vi "HFRR ADV v08.vi"() -> ()   [LabVIEW 2025] (continued)
                      frame #5 {
                        n2274 = local read "FILE"() -> (w3535:string)
                        n2275 = Concatenate Strings("File Name :" ("Content"), w3535) -> (w3536:string)
                        n2276 = local read "EVENT LOG"() -> (w3539:string)
                        n2277 = call "Event Log.vi"("Content"=w3536, "EVENT LOG"=w3539) -> ("EVENT LOG"=w3538:string)  [unwired: 8 in, 1 out]
                        n2278 = local write "EVENT LOG"(w3538) -> ()
                      }
                      frame #6 {
                        n2279 = Wait (ms)(milliseconds to wait=u32 50) -> ()  [unwired: 1 out]
                      }
                      frame #7 {
                        n2280 = local read "Batch Ref Num :"() -> (w3541:string)
                        n2281 = Concatenate Strings("Batch Ref No :" ("Content"), w3541) -> (w3542:string)
                        n2282 = local read "EVENT LOG"() -> (w3545:string)
                        n2283 = call "Event Log.vi"("Content"=w3542, "EVENT LOG"=w3545) -> ("EVENT LOG"=w3544:string)  [unwired: 8 in, 1 out]
                        n2284 = local write "EVENT LOG"(w3544) -> ()
                      }
                      frame #8 {
                        n2285 = Wait (ms)(milliseconds to wait=u32 50) -> ()  [unwired: 1 out]
                      }
                      frame #9 {
                        n2286 = local read "tested by"() -> (w3547:string)
                        n2287 = Concatenate Strings("Tested By :" ("Content"), w3547) -> (w3548:string)
                        n2288 = local read "EVENT LOG"() -> (w3551:string)
                        n2289 = call "Event Log.vi"("Content"=w3548, "EVENT LOG"=w3551) -> ("EVENT LOG"=w3550:string)  [unwired: 8 in, 1 out]
                        n2290 = local write "EVENT LOG"(w3550) -> ()
                      }
                      frame #10 {
                        n2291 = Wait (ms)(milliseconds to wait=u32 50) -> ()  [unwired: 1 out]
                      }
                      frame #11 {
                        n2292 = local read "TEST STANDARD"() -> (w3554:T4)
                        n2293 = case shown="\"ASTM D6079\", Default" w3554 {
                          tunnel: ["ASTM D6079" "ISO 12156" "CEC F-096-A-06" "Custom"] -> w3553
                          frame "ASTM D6079", Default {
                          }
                          frame "ISO 12156" {
                          }
                          frame "CEC F-096-A-06" {
                          }
                          frame "Custom" {
                          }
                        }
                        n2294 = Concatenate Strings("Test Standard :" ("Content"), w3553) -> (w3555:string)
                        n2295 = local read "EVENT LOG"() -> (w3558:string)
                        n2296 = call "Event Log.vi"("Content"=w3555, "EVENT LOG"=w3558) -> ("EVENT LOG"=w3557:string)  [unwired: 8 in, 1 out]
                        n2297 = local write "EVENT LOG"(w3557) -> ()
                      }
                      frame #12 {
                        n2298 = Wait (ms)(milliseconds to wait=u32 50) -> ()  [unwired: 1 out]
                      }
                      frame #13 {
                        n2299 = local read "Fuel Discription :"() -> (w3564:string)
                        n2300 = Concatenate Strings("Fuel Description :" ("Content"), w3564) -> (w3565:string)
                        n2301 = local read "EVENT LOG"() -> (w3568:string)
                        n2302 = call "Event Log.vi"("Content"=w3565, "EVENT LOG"=w3568) -> ("EVENT LOG"=w3567:string)  [unwired: 8 in, 1 out]
                        n2303 = local write "EVENT LOG"(w3567) -> ()
                      }
                      frame #14 {
                        n2304 = Wait (ms)(milliseconds to wait=u32 50) -> ()  [unwired: 1 out]
                      }
                      frame #15 {
                        n2305 = local read "Remarks :"() -> (w3570:string)
                        n2306 = Concatenate Strings("Remarks :" ("Content"), w3570) -> (w3571:string)
                        n2307 = local read "EVENT LOG"() -> (w3574:string)
                        n2308 = call "Event Log.vi"("Content"=w3571, "EVENT LOG"=w3574) -> ("EVENT LOG"=w3573:string)  [unwired: 8 in, 1 out]
                        n2309 = local write "EVENT LOG"(w3573) -> ()
                      }
                      frame #16 {
                        n2310 = Wait (ms)(milliseconds to wait=u32 50) -> ()  [unwired: 1 out]
                      }
                      frame #17 {
                        n2311 = local read "Operator ID"() -> (w3576:string)
                        n2312 = Concatenate Strings("Operator ID :" ("Content"), w3576) -> (w3578:string)
                        n2313 = local read "EVENT LOG"() -> (w3580:string)
                        n2314 = call "Event Log.vi"("Content"=w3578, "EVENT LOG"=w3580) -> ("EVENT LOG"=w3579:string)  [unwired: 8 in, 1 out]
                        n2315 = local write "EVENT LOG"(w3579) -> ()
                      }
                      frame #18 {
                        n2316 = Wait (ms)(milliseconds to wait=u32 50) -> ()  [unwired: 1 out]
                      }
                      frame #19 {
                        n2317 = disable-structure shown="Disabled" {
                          frame Disabled {
                            n2318 = local read "EVENT LOG"() -> (w3584:string)
                            n2319 = call "Event Log.vi"("Content"="Test Parameter", "EVENT LOG"=w3584) -> ("EVENT LOG"=w3583:string)  [unwired: 8 in, 1 out]
                            n2320 = local write "EVENT LOG"(w3583) -> ()
                          }
                          frame Enabled {
                          }
                        }
                      }
                      frame #20 {
                        n2321 = Wait (ms)(milliseconds to wait=u32 50) -> ()  [unwired: 1 out]
                      }
                      frame #21 {
                        n2322 = local read "Set Hz"() -> (w3588:dbl)
                        n2323 = Number To Fractional String(number=w3588, precision (6)=i16 2) -> (F-format string=w3587:string)  [unwired: 2 in]
                        n2324 = Concatenate Strings("Set Frequency [Hz] :" ("Content"), w3587) -> (w3590:string)
                        n2325 = local read "EVENT LOG"() -> (w3592:string)
                        n2326 = call "Event Log.vi"("Content"=w3590, "EVENT LOG"=w3592) -> ("EVENT LOG"=w3591:string)  [unwired: 8 in, 1 out]
                        n2327 = local write "EVENT LOG"(w3591) -> ()
                      }
                      frame #22 {
                        n2328 = Wait (ms)(milliseconds to wait=u32 50) -> ()  [unwired: 1 out]
                      }
                      frame #23 {
                        n2329 = local read "NORMAL LOAD"() -> (w3595:dbl)
                        n2330 = Number To Fractional String(number=w3595, precision (6)=i16 2) -> (F-format string=w3596:string)  [unwired: 2 in]
                        n2331 = Concatenate Strings("Applied Load [N] :" ("Content"), w3596) -> (w3598:string)
                        n2332 = local read "EVENT LOG"() -> (w3600:string)
                        n2333 = call "Event Log.vi"("Content"=w3598, "EVENT LOG"=w3600) -> ("EVENT LOG"=w3599:string)  [unwired: 8 in, 1 out]
                        n2334 = local write "EVENT LOG"(w3599) -> ()
                      }
                      frame #24 {
                        n2335 = Wait (ms)(milliseconds to wait=u32 50) -> ()  [unwired: 1 out]
                      }
                      frame #25 {
                        n2336 = local read "Set Strk"() -> (w3603:dbl)
                        n2337 = Number To Fractional String(number=w3603, precision (6)=i16 2) -> (F-format string=w3604:string)  [unwired: 2 in]
                        n2338 = Concatenate Strings("Set Stroke [mm] :" ("Content"), w3604) -> (w3606:string)
                        n2339 = local read "EVENT LOG"() -> (w3608:string)
                        n2340 = call "Event Log.vi"("Content"=w3606, "EVENT LOG"=w3608) -> ("EVENT LOG"=w3607:string)  [unwired: 8 in, 1 out]
                        n2341 = local write "EVENT LOG"(w3607) -> ()
                      }
                      frame #26 {
                        n2342 = Wait (ms)(milliseconds to wait=u32 50) -> ()  [unwired: 1 out]
                      }
                      frame #27 {
                        n2343 = local read "Set Temp"() -> (w3611:dbl)
                        n2344 = Number To Fractional String(number=w3611, precision (6)=i16 2) -> (F-format string=w3612:string)  [unwired: 2 in]
                        n2345 = Concatenate Strings("Set Temperature [deg C] :" ("Content"), w3612) -> (w3614:string)
                        n2346 = local read "EVENT LOG"() -> (w3616:string)
                        n2347 = call "Event Log.vi"("Content"=w3614, "EVENT LOG"=w3616) -> ("EVENT LOG"=w3615:string)  [unwired: 8 in, 1 out]
                        n2348 = local write "EVENT LOG"(w3615) -> ()
                      }
                      frame #28 {
                        n2349 = Wait (ms)(milliseconds to wait=u32 50) -> ()  [unwired: 1 out]
                      }
                      frame #29 {
                        n2350 = local read "Set Rh"() -> (w3619:dbl)
                        n2351 = Number To Fractional String(number=w3619, precision (6)=i16 2) -> (F-format string=w3620:string)  [unwired: 2 in]
                        n2352 = Concatenate Strings("Set Humidity [%RH] :" ("Content"), w3620) -> (w3622:string)
                        n2353 = local read "EVENT LOG"() -> (w3624:string)
                        n2354 = call "Event Log.vi"("Content"=w3622, "EVENT LOG"=w3624) -> ("EVENT LOG"=w3623:string)  [unwired: 8 in, 1 out]
                        n2355 = local write "EVENT LOG"(w3623) -> ()
                      }
                      frame #30 {
                        n2356 = Wait (ms)(milliseconds to wait=u32 50) -> ()  [unwired: 1 out]
                      }
                      frame #31 {
                        n2357 = local read "test time"() -> (w3627:dbl)
                        n2358 = Number To Fractional String(number=w3627, precision (6)=i16 1) -> (F-format string=w3628:string)  [unwired: 2 in]
                        n2359 = Concatenate Strings("Test Duration [mins] :" ("Content"), w3628) -> (w3630:string)
                        n2360 = local read "EVENT LOG"() -> (w3632:string)
                        n2361 = call "Event Log.vi"("Content"=w3630, "EVENT LOG"=w3632) -> ("EVENT LOG"=w3631:string)  [unwired: 8 in, 1 out]
                        n2362 = local write "EVENT LOG"(w3631) -> ()
                      }
                    }
                  }
                }
              }
            }
          }
        }
        n2363 = case shown="True" w2930 {
          frame False {
            n2364 = local write "tfalg"(0.0 ("tfalg")) -> ()
          }
          frame True {
            n2365 = local read "tfalg"() -> (w3075:dbl)
            n2366 = Equal?(x=w3075, y=0.0) -> (x = y?=w3076:bool)
            n2367 = case shown="True" w3076 {
              frame False {
              }
              frame True {
                n2368 = local read "Total No. of Tests"() -> (w3079:dbl)
                n2369 = local write "tfalg"(1.0 ("tfalg")) -> ()
                n2370 = local write "acq 2"(FALSE ("acq 2")) -> ()
                n2371 = Wait (ms)(milliseconds to wait=u32 200) -> ()  [unwired: 1 out]
                n2372 = Increment(x=w3079) -> (x+1=w3078:dbl)
                n2373 = local write "Total No. of Tests"(w3078) -> ()
              }
            }
          }
        }
        n2374 = local write "Test \nStatus"(w2936) -> ()
        n2375 = local write "st enable"(w2936) -> ()
        n2376 = local write "PWR"(w2936) -> ()
        n2377 = local write "Save"(w2936) -> ()
        n2378 = local read "Main Tab"() -> (w2893:T3)
        n2379 = case shown="True" w2917 {
          tunnel: [FALSE ("RUN") TRUE ("RUN")] -> w2916
          tunnel: [_ 1] -> w2909
          frame False {
          }
          frame True {
          }
        }
        n2380 = In Range and Coerce(upper limit=w2924, x=w2897, lower limit=w2923) -> (In Range?=w2915:bool)  [unwired: 1 out]
        n2381 = In Range and Coerce(upper limit=w2921, x=w2896, lower limit=w2922) -> (In Range?=w2913:bool)  [unwired: 1 out]
        n2382 = case shown="True" w2929 {
          frame False {
            n2383 = local read "Rt 3"() -> (w3057:bool)
            n2384 = case shown="True" w3057 {
              frame False {
              }
              frame True {
                n2385 = local write "Rt 3"(FALSE ("Rt 3")) -> ()
                n2386 = local write "Json End Flg"(TRUE ("Upld AR 2")) -> ()
              }
            }
            "Rt" <- TRUE ("Rt")
            "Rt 2" <- FALSE ("Rt")
          }
          frame True {
            n2387 = local read "Rt"() -> (w3064:bool)
            n2388 = local write "Rt 2"(TRUE ("Rt 2")) -> ()
            n2389 = case shown="True" w3064 {
              frame False {
              }
              frame True {
                w3065 = TRUE ("Upld AR 2")
                n2390 = local write "Rt"(FALSE ("Rt")) -> ()
                n2391 = local write "Upld AR"(w3065) -> ()
                n2392 = local write "Json St Flg"(w3065) -> ()
              }
            }
            "Rt 3" <- TRUE ("Rt 3")
          }
        }
        n2393 = case shown="True" w2915 {
          tunnel: [FALSE ("RUN") TRUE ("RUN")] -> w2914
          tunnel: [_ 2] -> w2908
          frame False {
          }
          frame True {
          }
        }
        n2394 = case shown="True" w2913 {
          tunnel: [FALSE ("RUN") TRUE ("RUN")] -> w2912
          tunnel: [_ 3] -> w2907
          frame False {
          }
          frame True {
          }
        }
        n2395 = case shown="\"Acquire\"" w2893 {
          tunnel: w2895 -> [_ w3126]
          frame Default {
            w3125 = 0.0 ("output")
            n2396 = local write "PID-out"(w3125) -> ()
            n2397 = local write "Frequency ( Hz )"(w3125) -> ()
          }
          frame "Acquire" {
            n2398 = stacked-sequence {
              frame #0 {
                n2399 = local read "Auto Start Test"() -> (w3128:bool)
                n2400 = case shown="False" w3128 {
                  tunnel: "RUN" -> [w3149 w3152]
                  tunnel: [w3149 w3151] -> w3129
                  frame False {
                  }
                  frame True {
                    n2401 = local read "Auto Start Temp"() -> (w3150:bool)
                    n2402 = Or(x=w3152, y=w3150) -> (x .or. y?=w3151:bool)
                  }
                }
                n2403 = local read "clk"() -> (w3148:dbl)
                n2404 = local read "Save"() -> (w3144:bool)
                n2405 = Equal?(x=w3148, y=0.0) -> (x = y?=w3145:bool)
                n2406 = And(x=w3145, y=w3144) -> (x .and. y?=w3146:bool)
                n2407 = Not(x="Engage") -> (.not. x?=w3135:bool)
                n2408 = case shown="True" w3129 {
                  tunnel: [w3160 w3178] -> w3131
                  frame False {
                    w3160 = 0.0
                    n2409 = local read "Auto Start Test"() -> (w3156:bool)
                    n2410 = local write "Reinit PID"(TRUE) -> ()
                    n2411 = local write "Start Time"(TRUE ("Start Time")) -> ()
                    n2412 = property on="Stroke" class="DigNum (strict)"("Visible"=TRUE) -> ()  [unwired: 2 in, 2 out]
                    n2413 = property on="Stroke 2" class="DigNum (strict)"("Visible"=FALSE) -> ()  [unwired: 2 in, 2 out]
                    n2414 = case shown="False" w3156 {
                      frame False {
                        n2415 = property on="Heater Button" class="Bool (strict)"("DisabledEnum"=T15."Enabled" ("Disabled")) -> ()  [unwired: 2 in, 2 out]
                        n2416 = property on="Humidity" class="Bool (strict)"("DisabledEnum"=T15."Enabled" ("Disabled")) -> ()  [unwired: 2 in, 2 out]
                      }
                      frame True {
                      }
                    }
                    n2417 = case shown="False" "TestCompFlg" {
                      frame False {
                        n2418 = local read "StartFlg"() -> (w3166:bool)
                        n2419 = case shown="True" w3166 {
                          frame False {
                          }
                          frame True {
                            n2420 = flat-sequence {
                              frame #0 {
                                n2421 = local read "EVENT LOG"() -> (w3168:string)
                                n2422 = call "Event Log.vi"("Content"="Test was interrupted", "EVENT LOG"=w3168) -> ("EVENT LOG"=w3169:string)  [unwired: 8 in, 1 out]
                                n2423 = local write "EVENT LOG"(w3169) -> ()
                              }
                              frame #1 {
                                w3170 = FALSE ("StartFlg")
                                n2424 = local write "Heater Button"(w3170) -> ()
                                n2425 = local write "StartFlg"(w3170) -> ()
                                n2426 = local write "Humidity"(w3170) -> ()
                              }
                            }
                          }
                        }
                      }
                      frame True {
                      }
                    }
                    n2427 = local write "String 14"("Test will autostart once parameters reach the set value." ("String 14")) -> ()
                    n2428 = local write "Old Pid Val"(w3160) -> ()
                  }
                  frame True {
                    n2429 = property on="Stroke 2" class="DigNum (strict)"("Visible"=TRUE) -> ()  [unwired: 2 in, 2 out]
                    n2430 = property on="Stroke" class="DigNum (strict)"("Visible"=FALSE) -> ()  [unwired: 2 in, 2 out]
                    n2431 = property on="STOP 2" class="Bool (strict)"("Disabled"=u8 2) -> ()  [unwired: 2 in, 2 out]
                    n2432 = local write "String 14"(" Running....." ("String 14")) -> ()
                    n2433 = property on="Heater Button" class="Bool (strict)"("DisabledEnum"=T15."Disabled and Grayed Out" ("Disabled")) -> ()  [unwired: 2 in, 2 out]
                    n2434 = property on="Humidity" class="Bool (strict)"("DisabledEnum"=T15."Disabled and Grayed Out" ("Disabled")) -> ()  [unwired: 2 in, 2 out]
                    n2435 = local read "PID Ref"() -> (w3189:bool)
                    n2436 = case shown="True" w3189 {
                      tunnel: [w3195 w3211] -> w3188
                      frame False {
                        n2437 = local read "Old Pid Val"() -> (w3195:dbl)
                      }
                      frame True {
                        n2438 = local read "Set Hz"() -> (w3204:dbl)
                        n2439 = local read "Frequency"() -> (w3215:dbl)
                        n2440 = Add(x=w3204, y=10.0) -> (x+y=w3213:dbl)
                        n2441 = Add(x=w3204, y=-10.0 ("Offset")) -> (x+y=w3222:dbl)
                        n2442 = Add(x=w3204, y=-10.0) -> (x+y=w3214:dbl)
                        n2443 = In Range and Coerce(upper limit=w3213, x=w3215, lower limit=w3214) -> (coerced(x)=w3203:dbl)  [unwired: 1 out]
                        n2444 = Or(x="Reinit PID", y="Reinit PID") -> (x .or. y?=w3212:bool)
                        n2445 = Multiply(x=w3222, y=0.1 ("Gain")) -> (x*y=w3201:dbl)
                        n2446 = local read "Elapsed time"() -> (w3208:dbl)
                        n2447 = local read "SPEED OUT:"() -> (w3223:dbl)
                        n2448 = Add(x=w3201, y=1.5) -> (x+y=w3199:dbl)
                        n2449 = call-poly <vilib>:"PID.vi"("reinitialize? (F)"=w3212, "output range"=cluster{"output high":dbl, "output low":dbl} {"output high"=1.0, "output low"=-1.0}, "PID gains"=T11 {"proportional gain (Kc)"=0.0005, "integral time (Ti, min)"=0.001, "derivative time (Td, min)"=0.0} ("Motor PID"), "process variable"=w3203, "setpoint"=w3204) -> ("output"=w3202:dbl)  [unwired: 5 in, 1 out]
                        n2450 = Multiply(x=w3199, y=w3223) -> (x*y=w3198:dbl)
                        n2451 = Greater?(x=w3208, y=0.05) -> (0:w3207:bool)
                        n2452 = case shown="True" w3207 {
                          tunnel: w3202 -> [_ w3225]
                          tunnel: [0.0 ("output") w3225] -> w3205
                          frame False {
                          }
                          frame True {
                            n2453 = local write "Reinit PID"(FALSE ("Reinit PID")) -> ()
                          }
                        }
                        n2454 = Multiply(x=w3198, y=0.8) -> (x*y=w3197:dbl)
                        n2455 = Add(x=w3197, y=w3205) -> (x+y=w3210:dbl)
                        n2456 = flat-sequence {
                          tunnel: [w3228] -> w3211
                          tunnel: w3210 -> [w3228]
                          frame #0 {
                            n2457 = local write "PID Ref"(FALSE ("PID Ref")) -> ()
                          }
                        }
                      }
                    }
                    "Old Pid Val" <- w3188
                    n2458 = case shown="False" "Start Time" {
                      selector: "Start Time" -> [_ w3191]
                      frame False {
                      }
                      frame True {
                        n2459 = Not(x=w3191) -> (.not. x?=w3190:bool)
                        n2460 = local write "Start Time"(w3190) -> ()
                        n2461 = local read "EVENT LOG"() -> (w3192:string)
                        n2462 = call "Event Log.vi"("Content"="Test in progress", "EVENT LOG"=w3192) -> ("EVENT LOG"=w3194:string)  [unwired: 8 in, 1 out]
                        n2463 = local write "EVENT LOG"(w3194) -> ()
                      }
                    }
                    n2464 = local read "Set Hz"() -> (w3185:dbl)
                    n2465 = call <vilib>:"Uniform White Noise Waveform.vi"() -> ("signal out"=w3184:waveform(dbl))  [unwired: 10 in, 1 out]
                    n2466 = local read "Freq"() -> (w3177:dbl)
                    n2467 = Add(x=w3185, y=w3184) -> (x+y=w3183:waveform(dbl))
                    n2468 = Multiply(x=w3183, y=ext 0.1) -> (x*y=w3179:waveform(ext))
                    n2469 = Multiply(x=w3177, y=0.9) -> (x*y=w3180:dbl)
                    n2470 = Add(x=w3179, y=w3180) -> (x+y=w3178:waveform(ext))
                    "StartFlg" <- TRUE ("StartFlg")
                  }
                }
                n2471 = case shown="True" w3146 {
                  frame False {
                  }
                  frame True {
                    n2472 = local write "clk"(10.0 ("clk")) -> ()
                    n2473 = Get Date/Time In Seconds() -> (seconds since 1Jan1904=w3231:timestamp)
                    n2474 = To Double Precision Float(number=w3231) -> (double precision float=w3229:dbl)
                    n2475 = local write "acq timer"(w3229) -> ()
                    n2476 = local write "act save time"(w3229) -> ()
                  }
                }
                n2477 = call "Elapsed Time"("Time Target (s)"="Countdown", "Reset"=w3135) -> ("Elapsed Time (s)"=w3140:dbl, "Time has Elapsed"=w3138:bool)  [unwired: 10 in, 6 out]
                "Countdown 2" <- w3140
                n2478 = Subtract(x=w3140, y=2.0) -> (x-y=w3143:dbl)
                n2479 = Less?(x=w3143, y="Countdown") -> (x < y?=w3141:bool)
                n2480 = And(x=w3141, y=w3138) -> (x .and. y?=w3137:bool)
                n2481 = case shown="True" w3137 {
                  frame False {
                  }
                  frame True {
                    (unwired) dbl[] [] ("History Data")
                    n2482 = local write "Engage"(FALSE ("Engage")) -> ()
                    n2483 = local write "RUN"(TRUE ("RUN")) -> ()
                    n2484 = local read "Humidity ( %RH )"() -> (→"Rh Before":dbl)
                  }
                }
                n2485 = local read "Test \nStatus"() -> (w3133:bool)
                n2486 = Select(t=w3131, s=w3133, f=0.0) -> (s? t:f=w3132:dbl)
                n2487 = local write "Frequency ( Hz )"(w3132) -> ()
                n2488 = local write "Freq"(w3132) -> ()
              }
              frame #1 {
                w3254 = 1000000.0 ("x")
                # "Elapsed time\ncof\nstroke\nAir temp\nTemp\nHumidity"
                # "acq timer\n\nact save time"
                # "convert to microseconds"
                n2489 = local read "COUNT"() -> (w3237:i32)
                n2490 = local read "Rate"() -> (w3250:dbl)
                n2491 = Divide(x=w3254, y=w3250) -> (x/y=w3255:dbl)
                n2492 = Greater Or Equal?(x=w3237, y=250) -> (x >= y?=w3236:bool)
                n2493 = Get Date/Time In Seconds() -> (seconds since 1Jan1904=w3257:timestamp)
                n2494 = case shown="True" w3236 {
                  frame False {
                    n2495 = local read "COUNT"() -> (w3258:i32)
                    n2496 = Increment(x=w3258) -> (x+1=w3259:i32)
                    n2497 = local write "COUNT"(w3259) -> ()
                  }
                  frame True {
                    n2498 = local write "COUNT"(0 ("COUNT")) -> ()
                  }
                }
                n2499 = local read "Samplingtime 2"() -> (w3235:dbl)
                n2500 = local read "act save time"() -> (w3252:dbl)
                n2501 = Divide(x=w3255, y=w3254) -> (x/y=w3253:dbl)
                n2502 = To Double Precision Float(number=w3257) -> (double precision float=w3246:dbl)
                n2503 = Add(x=w3252, y=w3235) -> (x+y=w3251:dbl)
                n2504 = local read "acq timer"() -> (w3256:dbl)
                n2505 = local read "COUNT"() -> (w3239:i32)
                n2506 = Greater Or Equal?(x=w3246, y=w3251) -> (x >= y?=w3234:bool)
                n2507 = Multiply(x=w3253, y=w3239) -> (x*y=w3245:dbl)
                n2508 = Subtract(x=w3246, y=w3256) -> (x-y=w3248:dbl)
                n2509 = local read "Save"() -> (w3249:bool)
                n2510 = Add(x=w3248, y=w3245) -> (x+y=w3232:dbl)
                "Elapsed time 3" <- w3232
                n2511 = And(x=w3234, y=w3249) -> (x .and. y?=w3247:bool)
                n2512 = Divide(x=w3232, y=60.0) -> (x/y=w3243:dbl)
                n2513 = local read "Test \nStatus"() -> (w3233:bool)
                n2514 = local read "clk"() -> (w3240:dbl)
                n2515 = Equal?(x=w3240, y=10.0) -> (x = y?=w3242:bool)
                n2516 = case shown="True" w3247 {
                  tunnel: w3246 -> [_ w3353]
                  tunnel: [FALSE ("Boolean 2") TRUE ("Boolean 2")] -> _
                  frame False {
                  }
                  frame True {
                    w3300 = ";" ("Substring")
                    # "Pid out/\nFreq response value"
                    n2517 = local write "act save time"(w3353) -> ()
                    n2518 = local read "FILE"() -> (w3294:string)
                    n2519 = call "file check.vi"("file name in"=w3294) -> ("error out"=w3297:errorcluster, "file name out"=w3292:string)  [unwired: 9 in]
                    n2520 = call "FILE PATH CREATION.vi"("error in"=w3297, "FILE NAME :"=w3292) -> ("FILE OUT"=w3295:path)  [unwired: 8 in, 1 out]
                    n2521 = Concatenate Strings(w3292, ".dgf" ("Substring")) -> (w3296:string)
                    n2522 = local read "Set Strk"() -> (w3324:dbl)
                    n2523 = local read "Stroke"() -> (w3315:dbl)
                    n2524 = local read "FF 2"() -> (w3311:dbl)
                    "Frictional Force ( N )" <- w3311
                    "Frictional Force ( N )" <- w3311
                    n2525 = Build Path(base path=w3295, name or relative path=w3296) -> (appended path=w3291:path)
                    n2526 = local write "FF 3"(w3311) -> ()
                    n2527 = Subtract(x=w3315, y=w3324) -> (x-y=w3321:dbl)
                    n2528 = local read "COF 2"() -> (w3306:dbl)
                    "cof" <- w3306
                    "Coefficient of Friction" <- w3306
                    "COF 4" <- w3306
                    "Coefficient of Friction" <- w3306
                    n2529 = local write "COF 3"(w3306) -> ()
                    n2530 = Multiply(x=w3321, y=0.05) -> (x*y=w3323:dbl)
                    n2531 = local read "TEMP"() -> (w3310:dbl)
                    "Temp" <- w3310
                    "Temperature ( Deg C )" <- w3310
                    n2532 = Add(x=w3323, y=w3324) -> (x+y=w3304:dbl)
                    "Stroke Ln" <- w3304
                    "Disp" <- w3304
                    n2533 = local read "ecr"() -> (w3307:dbl)
                    "ecr 2" <- w3307
                    "Electrical Contact Resistance ( % )" <- w3307
                    "ecr 4" <- w3307
                    n2534 = local read "Humidity ( %RH )"() -> (w3309:dbl)
                    "Humidity ( %RH )" <- w3309
                    "Humidity ( %RH )" <- w3309
                    n2535 = local read "Frequency ( Hz )"() -> (w3317:dbl)
                    n2536 = local read "Elapsed time"() -> (w3346:dbl)
                    n2537 = local read "AIR TEMP"() -> (w3314:dbl)
                    n2538 = local write "ecr 3"(w3307) -> ()
                    n2539 = local read "PID-out"() -> (w3320:dbl)
                    n2540 = local write "Temperature ( Deg C )"(w3310) -> ()
                    n2541 = local write "Electrical Contact Resistance ( % )"(w3307) -> ()
                    n2542 = Number To Fractional String(number=w3304, width (-)=i16 9 ("precision (6)"), precision (6)=i16 6) -> (F-format string=w3339:string)  [unwired: 1 in]
                    n2543 = Number To Fractional String(number=w3314, width (-)=i16 9 ("precision (6)"), precision (6)=i16 3) -> (F-format string=w3338:string)  [unwired: 1 in]
                    n2544 = Number To Fractional String(number=w3310, width (-)=i16 9 ("precision (6)"), precision (6)=i16 3) -> (F-format string=w3335:string)  [unwired: 1 in]
                    n2545 = Number To Fractional String(number=w3309, width (-)=i16 9 ("precision (6)"), precision (6)=i16 3) -> (F-format string=w3332:string)  [unwired: 1 in]
                    n2546 = Number To Fractional String(number=w3307, width (-)=i16 9 ("precision (6)"), precision (6)=i16 3) -> (F-format string=w3329:string)  [unwired: 1 in]
                    n2547 = Number To Fractional String(number=w3320, width (-)=i16 9 ("precision (6)"), precision (6)=i16 3) -> (F-format string=w3325:string)  [unwired: 1 in]
                    n2548 = Number To Fractional String(number=w3317, width (-)=i16 9 ("precision (6)"), precision (6)=i16 3) -> (F-format string=w3316:string)  [unwired: 1 in]
                    n2549 = Number To Fractional String(number=w3306, width (-)=i16 9 ("precision (6)"), precision (6)=i16 6) -> (F-format string=w3347:string)  [unwired: 1 in]
                    n2550 = Number To Fractional String(number=w3346, width (-)=i16 14 ("precision (6)"), precision (6)=i16 3) -> (F-format string=w3348:string)  [unwired: 1 in]
                    n2551 = Bundle("y"=1.02, w3304, "y"=0.98) -> (w3308:cluster{"y":dbl, dbl, "y":dbl})  [unwired: 1 in]
                    n2552 = Number To Fractional String(number="Ambient Humidity :", width (-)=i16 9 ("precision (6)"), precision (6)=i16 6) -> (F-format string=w3298:string)  [unwired: 1 in]
                    n2553 = local read "RUN"() -> (w3305:bool)
                    n2554 = case shown="True" w3305 {
                      tunnel: w3308 -> [_ w3358]
                      tunnel: w3304 -> [_ w3357]
                      tunnel: w3304 -> [_ w3356]
                      tunnel: w3304 -> [_ w3355]
                      frame False {
                      }
                      frame True {
                        "Stroke ( mm )" <- w3358
                        "Stroke ( mm )" <- w3358
                        "Stroke 4" <- w3357
                        "Stroke 3" <- w3356
                        "Stroke 2" <- w3355
                      }
                    }
                    n2555 = Concatenate Strings(w3348, w3300, w3347, w3300, w3339, w3300, w3338, w3300, w3335, w3300, w3332, w3300, w3329, w3300, w3325, w3300, w3316, w3300, w3298, "\r") -> (w3345:string)
                    n2556 = call <vilib>:"Write Characters To File.vi"("append to file? (new file:F)"=TRUE, "character string"=w3345, "file path (dialog if empty)"=w3291) -> ()  [unwired: 2 in, 1 out]
                    "refresh flag" <- TRUE ("refresh flag")
                  }
                }
                n2557 = case shown="True" w3233 {
                  tunnel: w3243 -> [_ w3267]
                  tunnel: w3248 -> [_ w3277]
                  tunnel: [0.0 w3273] -> _
                  tunnel: w3242 -> [_ w3272]
                  tunnel: [0.0 w3271] -> _
                  tunnel: w3232 -> [_ w3271]
                  tunnel: w3246 -> [w3262 _]
                  frame False {
                    n2558 = local write "acq timer"(w3262) -> ()
                    n2559 = local write "Test Duration Status"(0.0 ("Test Duration Status")) -> ()
                  }
                  frame True {
                    n2560 = local read "Set Hz"() -> (w3274:dbl)
                    n2561 = local write "Elapsed time"(w3267) -> ()
                    n2562 = local read "test time"() -> (w3266:dbl)
                    n2563 = Multiply(x=w3277, y=w3274) -> (x*y=w3276:dbl)
                    n2564 = case shown="False" w3272 {
                      tunnel: w3276 -> [w3278 _]
                      tunnel: [w3278 1.0] -> w3273
                      frame False {
                        n2565 = local write "Cycles elapsed"(w3278) -> ()
                      }
                      frame True {
                      }
                    }
                    n2566 = Greater?(x=w3267, y=w3266) -> (0:w3275:bool)
                    n2567 = Subtract(x=w3266, y=w3267) -> (x-y=w3265:dbl)
                    "time" <- w3265
                    n2568 = local write "Time Remaining"(w3265) -> ()
                    n2569 = local write "Remaining Time"(w3265) -> ()
                    n2570 = case shown="True" w3275 {
                      frame False {
                      }
                      frame True {
                        n2571 = local write "Humidity"(FALSE ("Humidity")) -> ()
                        n2572 = local write "RUN"(FALSE ("OK Button 2")) -> ()
                        n2573 = local write "Heater Button"(FALSE ("Heater Button")) -> ()
                        n2574 = local write "Auto Start Test"(FALSE ("Auto Start Test")) -> ()
                        n2575 = local write "TestCompFlg"(TRUE ("StpFlg")) -> ()
                        n2576 = local read "Humidity ( %RH )"() -> (→"Rh After":dbl)
                        n2577 = property on="STOP 2" class="Bool (strict)"("Disabled"=u8 0) -> ()  [unwired: 2 in, 2 out]
                        n2578 = local read "EVENT LOG"() -> (w3284:string)
                        n2579 = call "Event Log.vi"("Content"="Test Completed", "EVENT LOG"=w3284) -> ("EVENT LOG"=w3283:string)  [unwired: 8 in, 1 out]
                        n2580 = local write "EVENT LOG"(w3283) -> ()
                      }
                    }
                    n2581 = Divide(x=w3267, y=w3266) -> (x/y=w3270:dbl)
                    n2582 = Multiply(x=w3270, y=100.0) -> (x*y=w3268:dbl)
                    n2583 = local write "Test Duration Status"(w3268) -> ()
                  }
                }
              }
              frame #2 {
                n2584 = case shown="True" "Heater Button" {
                  tunnel: [0.0 ("output") w3382] -> w3359
                  frame False {
                    w3362 = TRUE ("tmpchk")
                    n2585 = local read "TEMP"() -> (w3363:dbl)
                    n2586 = local write "Temp ini"(w3363) -> ()
                    n2587 = local write "Reset 4"(w3362) -> ()
                    n2588 = local write "tmpchk"(w3362) -> ()
                    n2589 = local write "reinit"(TRUE ("reinit")) -> ()
                    n2590 = local write "manual temp log"(TRUE ("manual temp log")) -> ()
                  }
                  frame True {
                    # "Logic to turn off\nthe heater when \ntemp is not rising.\nTime - 60 sec\nDelta t- 5°c"
                    n2591 = local read "Temp ini"() -> (w3370:dbl)
                    n2592 = local read "Auto Start Test"() -> (w3366:bool)
                    n2593 = Less?(x=w3370, y=53.0) -> (x < y?=w3368:bool)
                    n2594 = case shown="False" w3366 {
                      frame False {
                        n2595 = local read "Set Temp"() -> (w3393:dbl)
                        n2596 = local read "TEMP"() -> (w3392:dbl)
                        n2597 = Subtract(x=w3393, y=w3392) -> (x-y=w3391:dbl)
                        n2598 = Absolute Value(x=w3391) -> (abs(x)=w3390:dbl)
                        n2599 = Less?(x=w3390, y=0.5) -> (x < y?=w3388:bool)
                        n2600 = case shown="True" w3388 {
                          tunnel: "manual temp log" -> [_ w3394]
                          frame False {
                          }
                          frame True {
                            n2601 = case shown="True" w3394 {
                              selector: w3394 -> [_ w3395]
                              frame False {
                              }
                              frame True {
                                # "#Event log"
                                n2602 = Not(x=w3395) -> (.not. x?=w3396:bool)
                                n2603 = local write "manual temp log"(w3396) -> ()
                                n2604 = local read "EVENT LOG"() -> (w3399:string)
                                n2605 = call "Event Log.vi"("Content"="Target Temperature reached", "EVENT LOG"=w3399) -> ("EVENT LOG"=w3398:string)  [unwired: 8 in, 1 out]
                                n2606 = local write "EVENT LOG"(w3398) -> ()
                              }
                            }
                          }
                        }
                      }
                      frame True {
                        n2607 = local write "manual temp log"(TRUE ("manual temp log")) -> ()
                      }
                    }
                    n2608 = And(x="tmpchk", y=w3368) -> (x .and. y?=w3371:bool)
                    n2609 = case shown="True" w3371 {
                      frame False {
                      }
                      frame True {
                        n2610 = call "Elapsed Time8"("Time Target (s)"=300.0, "Reset"="Reset 4") -> ("Time has Elapsed"=w3401:bool)  [unwired: 10 in, 7 out]
                        n2611 = flat-sequence {
                          tunnel: w3401 -> [_]
                          frame #0 {
                            n2612 = local write "Reset 4"(FALSE ("Reset 4")) -> ()
                          }
                        }
                        n2613 = case shown="True" w3401 {
                          frame False {
                          }
                          frame True {
                            n2614 = local read "Temp ini"() -> (w3408:dbl)
                            n2615 = Add(x=w3408, y=5.0) -> (x+y=w3406:dbl)
                            n2616 = local read "TEMP"() -> (w3409:dbl)
                            n2617 = Greater?(x=w3409, y=w3406) -> (0:w3407:bool)
                            n2618 = case shown="False" w3407 {
                              frame False {
                                n2619 = local write "Heater Button"(FALSE ("Heater Button")) -> ()
                              }
                              frame True {
                                n2620 = local write "tmpchk"(FALSE ("tmpchk")) -> ()
                              }
                            }
                          }
                        }
                      }
                    }
                    n2621 = local read "Set Temp"() -> (w3379:dbl)
                    n2622 = local read "TEMP"() -> (w3373:dbl)
                    n2623 = call-poly <vilib>:"PID.vi"("reinitialize? (F)"="reinit", "output range"="output range", "dt (s)"=-1.0, "PID gains"="Temp PID gains", "process variable"=w3373, "setpoint"=w3379) -> ("output"=w3376:dbl)  [unwired: 4 in, 1 out]
                    n2624 = Subtract(x=w3379, y=w3373) -> (x-y=w3381:dbl)
                    n2625 = Add(x=w3379, y=0.5) -> (x+y=w3377:dbl)
                    n2626 = Greater Or Equal?(x=w3373, y=w3377) -> ()  [unwired: 1 out]
                    n2627 = Select(t=0.0, s=FALSE, f=w3376) -> (s? t:f=w3375:dbl)
                    "PID output" <- w3375
                    n2628 = flat-sequence {
                      tunnel: w3375 -> [w3412]
                      tunnel: [w3412] -> w3382
                      frame #0 {
                        n2629 = local write "reinit"(FALSE ("reinit")) -> ()
                      }
                    }
                    n2630 = Bundle(w3381, "output"=w3375, "TEMP"=w3373) -> (→"gTEMP 3":cluster{dbl, "output":dbl, "TEMP":dbl})  [unwired: 1 in]
                  }
                }
                "PID-out" <- w3359
              }
              frame #3 {
                n2631 = local read "TEMP"() -> (w3414:dbl)
                n2632 = Greater Or Equal?(x=w3414, y="Set Temp 2") -> (x >= y?=w3419:bool)
                n2633 = case shown="True" w3419 {
                  tunnel: [FALSE TRUE] -> w3417
                  frame False {
                  }
                  frame True {
                  }
                }
                "Status 13" <- w3417
                n2634 = And(x=w3417, y="trip1 8") -> (x .and. y?=w3416:bool)
                n2635 = case shown="True" w3416 {
                  frame False {
                  }
                  frame True {
                    w3420 = FALSE ("OK Button 2")
                    n2636 = local write "RUN"(w3420) -> ()
                    n2637 = local write "Heater Button"(w3420) -> ()
                  }
                }
              }
            }
            n2638 = case shown="False" w3126 {
              frame False {
                n2639 = disable-structure shown="Enabled" {
                  frame Enabled {
                    n2640 = stacked-sequence {
                      frame #0 {
                        n2641 = local write "RUN"(FALSE ("OK Button 2")) -> ()
                      }
                      frame #1 {
                      }
                    }
                  }
                  frame Disabled {
                  }
                }
              }
              frame True {
              }
            }
          }
        }
        n2642 = local read "airtempflg"() -> (w2918:bool)
        n2643 = Or(x=w2918, y=w2916) -> (x .or. y?=w2919:bool)
        n2644 = Insert Into Array(array=string[] ["Air Temperature has reached set value,", "Humidity has reached set value,", "Sample Temperaturehas reached set value,", ""], index=0, new element="") -> (w2904:string[])
        n2645 = Build Array(w2909, w2908, w2907) -> (w2905:i32[])
        n2646 = disable-structure shown="Disabled" {
          disable-tunnel: w2919 -> [w2996 _]
          disable-tunnel: w2914 -> [w2995 _]
          disable-tunnel: w2912 -> [w2994 _]
          frame Disabled {
            n2647 = Compound Arithmetic op=AND(w2996, w2995, w2994) -> ()  [unwired: 1 out]
            n2648 = case shown="True" {
              selector: _ -> [_ _]
              frame False {
              }
              frame True {
                w2997 = FALSE ("autostrtflg")
                n2649 = local write "RUN"(TRUE ("RUN")) -> ()
                n2650 = local write "autostrtflg"(w2997) -> ()
                n2651 = local write "autostart"(w2997) -> ()
                n2652 = local write "String 14"(" Running....." ("String 14")) -> ()
              }
            }
          }
          frame Enabled {
          }
        }
        n2653 = for {
          tunnel: w2905 -> [w3047] mode=indexing
          tunnel: w2904 -> [w3046]
          shift-right: [w3043] -> w2903
          shift-left: "" -> [w3045]
          n2654 = Index Array(array=w3046, index=w3047) -> (element=w3044:string)
          n2655 = Concatenate Strings(w3044, w3045) -> (w3043:string)
        }
        n2656 = local write "autostart 2"(w2903) -> ()
        n2657 = local read "Reset Graph"() -> (w2892:bool)
        n2658 = case shown="True" w2892 {
          selector: w2892 -> [_ w2946]
          frame False {
          }
          frame True {
            w2960 = 0.0 ("X Scale.Range:Maximum")
            n2659 = Not(x=w2946) -> (.not. x?=w2945:bool)
            n2660 = local write "Reset Graph"(w2945) -> ()
            n2661 = property on="Electrical Contact Resistance ( % )" class="WFChart (strict)"("XScale.Maximum"=600.0 ("X Scale.Range:Maximum"), "XScale.Minimum"=0.0 ("X Scale.Range:Minimum"), "YScale.Maximum"=100.0 ("Y Scale.Range:Maximum"), "YScale.Minimum"=0.0 ("Y Scale.Range:Minimum")) -> ()  [unwired: 2 in, 2 out]
            n2662 = property on="Frictional Force ( N )" class="WFChart (strict)"("XScale.Maximum"=600.0 ("X Scale.Range:Maximum"), "XScale.Minimum"=0.0 ("X Scale.Range:Minimum"), "YScale.Maximum"=100.0 ("Y Scale.Range:Maximum"), "YScale.Minimum"=0.0 ("Y Scale.Range:Minimum")) -> ()  [unwired: 2 in, 2 out]
            n2663 = property on="Temperature ( Deg C )" class="WFChart (strict)"("XScale.Maximum"=600.0 ("X Scale.Range:Maximum"), "XScale.Minimum"=0.0 ("X Scale.Range:Minimum"), "YScale.Maximum"=100.0 ("Y Scale.Range:Maximum"), "YScale.Minimum"=0.0 ("Y Scale.Range:Minimum")) -> ()  [unwired: 2 in, 2 out]
            n2664 = property on="Humidity ( %RH )" class="WFChart (strict)"("XScale.Maximum"=600.0 ("X Scale.Range:Maximum"), "XScale.Minimum"=0.0 ("X Scale.Range:Minimum"), "YScale.Maximum"=100.0 ("Y Scale.Range:Maximum"), "YScale.Minimum"=0.0 ("Y Scale.Range:Minimum")) -> ()  [unwired: 2 in, 2 out]
            n2665 = property on="Stroke ( mm )" class="WFChart (strict)"("XScale.Maximum"=600.0 ("X Scale.Range:Maximum"), "XScale.Minimum"=0.0 ("X Scale.Range:Minimum"), "YScale.Maximum"=100.0 ("Y Scale.Range:Maximum"), "YScale.Minimum"=0.0 ("Y Scale.Range:Minimum")) -> ()  [unwired: 2 in, 2 out]
            n2666 = property on="Coefficient of Friction" class="WFChart (strict)"("XScale.Maximum"=600.0 ("X Scale.Range:Maximum"), "XScale.Minimum"=0.0 ("X Scale.Range:Minimum"), "YScale.Maximum"=100.0 ("Y Scale.Range:Maximum"), "YScale.Minimum"=0.0 ("Y Scale.Range:Minimum")) -> ()  [unwired: 2 in, 2 out]
            n2667 = property on="Electrical Contact Resistance ( % )" class="WFChart (strict)"("XScale.Minimum"=0.0 ("X Scale.Range:Minimum"), "XScale.Maximum"=600.0 ("X Scale.Range:Maximum"), "YScale.Minimum"=0.0 ("Y Scale.Range:Minimum"), "YScale.Maximum"=100.0 ("Y Scale.Range:Maximum")) -> ()  [unwired: 2 in, 2 out]
            n2668 = property on="Temperature ( Deg C )" class="WFChart (strict)"("XScale.Minimum"=0.0 ("X Scale.Range:Minimum"), "XScale.Maximum"=600.0 ("X Scale.Range:Maximum"), "YScale.Minimum"=0.0 ("Y Scale.Range:Minimum"), "YScale.Maximum"=100.0 ("Y Scale.Range:Maximum")) -> ()  [unwired: 2 in, 2 out]
            n2669 = property on="Coefficient of Friction" class="WFChart (strict)"("XScale.Minimum"=0.0 ("X Scale.Range:Minimum"), "XScale.Maximum"=600.0 ("X Scale.Range:Maximum"), "YScale.Maximum"=1.0 ("X Scale.Range:Minimum"), "YScale.Minimum"=0.0 ("X Scale.Range:Minimum")) -> ()  [unwired: 2 in, 2 out]
            n2670 = property on="Frictional Force ( N )" class="WFChart (strict)"("XScale.Maximum"=600.0 ("X Scale.Range:Maximum"), "XScale.Minimum"=w2960, "YScale.Maximum"=10.0 ("Y Scale.Range:Maximum"), "YScale.Minimum"=w2960) -> ()  [unwired: 2 in, 2 out]
            n2671 = property on="Stroke ( mm )" class="WFChart (strict)"("XScale.Maximum"=600.0 ("X Scale.Range:Maximum"), "XScale.Minimum"=0.0 ("X Scale.Range:Minimum"), "YScale.Maximum"=100.0 ("Y Scale.Range:Maximum"), "YScale.Minimum"=0.0 ("Y Scale.Range:Minimum")) -> ()  [unwired: 2 in, 2 out]
            n2672 = property on="Humidity ( %RH )" class="WFChart (strict)"("XScale.Maximum"=600.0 ("X Scale.Range:Maximum"), "XScale.Minimum"=0.0 ("X Scale.Range:Minimum"), "YScale.Maximum"=100.0 ("Y Scale.Range:Maximum"), "YScale.Minimum"=0.0 ("Y Scale.Range:Minimum")) -> ()  [unwired: 2 in, 2 out]
          }
        }
      }
      frame "Compare Files" {
        # "Elapsed time\ncof\nstroke\nAir temp\nTemp\nHumidity"
        n2673 = case shown="True" "RSTV1 2" {
          frame False {
          }
          frame True {
            n2674 = property on="Humidity ( %RH )" class="XYGraph (strict)"("Y Scale.Display Format:Precision"=u8 0 ("Y Scale.Format & Precision:Precision")) -> ()  [unwired: 2 in, 2 out]
            n2675 = property on="Humidity ( %RH )" class="XYGraph (strict)"("X Scale.Range:Minimum"=0.0, "X Scale.Range:Maximum"=75.0, "Y Scale.Range:Minimum"=48.0, "Y Scale.Range:Maximum"=58.0) -> ()  [unwired: 2 in, 2 out]
          }
        }
        n2676 = case shown="True" "RST CP 2" {
          frame False {
          }
          frame True {
            n2677 = property on="XY Graph 13" class="XYGraph (strict)"("Y Scale.Display Format:Precision"=u8 0 ("Y Scale.Format & Precision:Precision")) -> ()  [unwired: 2 in, 2 out]
            n2678 = property on="XY Graph 13" class="XYGraph (strict)"("X Scale.Range:Minimum"=0.0, "X Scale.Range:Maximum"=75.0, "Y Scale.Range:Minimum"=0.0, "Y Scale.Range:Maximum"=100.0) -> ()  [unwired: 2 in, 2 out]
          }
        }
        n2679 = case shown="True" "RST CP" {
          frame False {
          }
          frame True {
            n2680 = property on="Sample Temperature ( °C )" class="XYGraph (strict)"("Y Scale.Display Format:Precision"=u8 2 ("Y Scale.Format & Precision:Precision")) -> ()  [unwired: 2 in, 2 out]
            n2681 = property on="Sample Temperature ( °C )" class="XYGraph (strict)"("X Scale.Range:Minimum"=0.0, "X Scale.Range:Maximum"=75.0, "Y Scale.Range:Minimum"=58.0, "Y Scale.Range:Maximum"=62.0) -> ()  [unwired: 2 in, 2 out]
          }
        }
        n2682 = case shown="True" "RSTV1 3" {
          frame False {
          }
          frame True {
            n2683 = property on="Air Temperature  ( °C )" class="XYGraph (strict)"("Y Scale.Display Format:Precision"=u8 2 ("Y Scale.Format & Precision:Precision")) -> ()  [unwired: 2 in, 2 out]
            n2684 = property on="Air Temperature  ( °C )" class="XYGraph (strict)"("X Scale.Range:Minimum"=0.0 ("Y Scale.Range:Minimum"), "X Scale.Range:Maximum"=75.0 ("Y Scale.Range:Maximum"), "Y Scale.Range:Minimum"=20.0 ("X Scale.Range:Minimum"), "Y Scale.Range:Maximum"=26.0 ("X Scale.Range:Maximum")) -> ()  [unwired: 2 in, 2 out]
          }
        }
        n2685 = case shown="True" "RSTV1 4" {
          frame False {
          }
          frame True {
            n2686 = property on="Stroke ( mm )" class="XYGraph (strict)"("Y Scale.Display Format:Precision"=u8 2 ("Y Scale.Format & Precision:Precision")) -> ()  [unwired: 2 in, 2 out]
            n2687 = property on="Stroke ( mm )" class="XYGraph (strict)"("X Scale.Range:Minimum"=0.0 ("Y Scale.Range:Maximum"), "X Scale.Range:Maximum"=75.0 ("X Scale.Range:Minimum"), "Y Scale.Range:Minimum"=0.98, "Y Scale.Range:Maximum"=1.02) -> ()  [unwired: 2 in, 2 out]
          }
        }
        n2688 = case shown="True" "rstv2" {
          frame False {
          }
          frame True {
            n2689 = property on="Coefficient Of Friction" class="XYGraph (strict)"("Y Scale.Display Format:Precision"=u8 3 ("Y Scale.Format & Precision:Precision")) -> ()  [unwired: 2 in, 2 out]
            n2690 = property on="Coefficient Of Friction" class="XYGraph (strict)"("X Scale.Range:Minimum"=0.0 ("Y Scale.Range:Maximum"), "X Scale.Range:Maximum"=75.0, "Y Scale.Range:Minimum"=0.0, "Y Scale.Range:Maximum"=1.0 ("X Scale.Range:Minimum")) -> ()  [unwired: 2 in, 2 out]
          }
        }
        n2691 = case shown="True" "RST CP 3" {
          frame False {
          }
          frame True {
            n2692 = property on="Air Temp ( °C ) vs Humidity ( % RH )" class="XYGraph (strict)"("X Scale.Range:Minimum"=18.0, "X Scale.Range:Maximum"=28.0 ("X Scale.Range:Minimum"), "Y Scale.Range:Minimum"=30.0 ("X Scale.Range:Minimum"), "Y Scale.Range:Maximum"=70.0 ("X Scale.Range:Minimum")) -> ()  [unwired: 2 in, 2 out]
          }
        }
        n2693 = case shown="True" "OPEN 1" {
          frame False {
          }
          frame True {
            (unwired) 0  # existing file
            w3685 = "Choose a datalog file to open"  # prompt
            n2694 = local write "OPEN 1"(FALSE ("OPEN 1")) -> ()
            n2695 = String To Path(string="C:\\LAB-IQ\\Data\\") -> (path=w3670:path)
            n2696 = File Dialog(6:"*.dgf" ("pattern"), 7:w3685, 11:w3670) -> (0:w3668:errorcluster, 3:w3676:path)  [unwired: 4 in, 2 out]
            n2697 = Unbundle(w3668) -> ()  [unwired: 3 out]
            n2698 = Strip Path(path=w3676) -> (name=w3675:string)  [unwired: 1 out]
            n2699 = Path To String(path=w3676) -> (string=w3671:string)
            "string1" <- w3671
            n2700 = Match Pattern(string=w3675, regular expression=".dgf") -> (before substring=→"String Control":string)  [unwired: 1 in, 3 out]
            n2701 = Match Pattern(string=w3671, regular expression=".dgf" ("substring (\"\")")) -> (before substring=w3681:string)  [unwired: 1 in, 3 out]
            n2702 = Concatenate Strings(w3681, ".duf" ("Substring")) -> (w3677:string)
            n2703 = String To Path(string=w3677) -> (path=w3682:path)
            n2704 = call <vilib>:"Read Characters From File.vi"("file path (dialog if empty)"=w3682, "start of read offset (chars.:0)"=60 ("start of read offset (chars.: 0)")) -> ("character string"=→"String Control 2":string)  [unwired: 4 in, 3 out]
          }
        }
        n2705 = case shown="True" "OPEN 2" {
          frame False {
          }
          frame True {
            (unwired) 0  # existing file
            w3703 = "Choose a datalog file to open"  # prompt
            n2706 = local write "OPEN 2"(FALSE ("OPEN 1")) -> ()
            n2707 = String To Path(string="C:\\LAB-IQ\\Data\\") -> (path=w3688:path)
            n2708 = File Dialog(6:"*.dgf" ("pattern"), 7:w3703, 11:w3688) -> (0:w3686:errorcluster, 3:w3694:path)  [unwired: 4 in, 2 out]
            n2709 = Unbundle(w3686) -> ()  [unwired: 3 out]
            n2710 = Strip Path(path=w3694) -> (name=w3692:string)  [unwired: 1 out]
            n2711 = Path To String(path=w3694) -> (string=w3689:string)
            "string1 2" <- w3689
            n2712 = Match Pattern(string=w3692, regular expression=".dgf") -> (before substring=→"String Control 3":string)  [unwired: 1 in, 3 out]
            n2713 = Match Pattern(string=w3689, regular expression=".dgf" ("substring (\"\")")) -> (before substring=w3700:string)  [unwired: 1 in, 3 out]
            n2714 = Concatenate Strings(w3700, ".duf" ("Substring")) -> (w3697:string)
            n2715 = String To Path(string=w3697) -> (path=w3695:path)
            n2716 = call <vilib>:"Read Characters From File.vi"("file path (dialog if empty)"=w3695, "start of read offset (chars.:0)"=60 ("start of read offset (chars.: 0)")) -> ("character string"=→"String Control 4":string)  [unwired: 4 in, 3 out]
          }
        }
        n2717 = case shown="True" "OPEN 3" {
          frame False {
          }
